vi "S2C_ExeScriptNextStep.vi"(8 "Error In":errorcluster, 11 "Q-Ref":refnum<queue>) -> (0 "Error Out":errorcluster)   [LabVIEW 2015]
doc: "Advances the executable script to the next step."
uses:
  Globals/S2C_Globals.vi
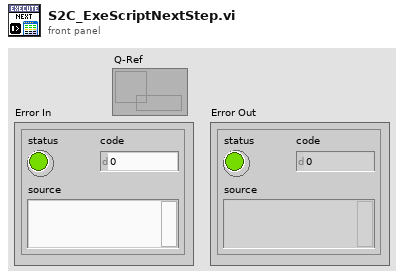
[diagram p1: front panel]
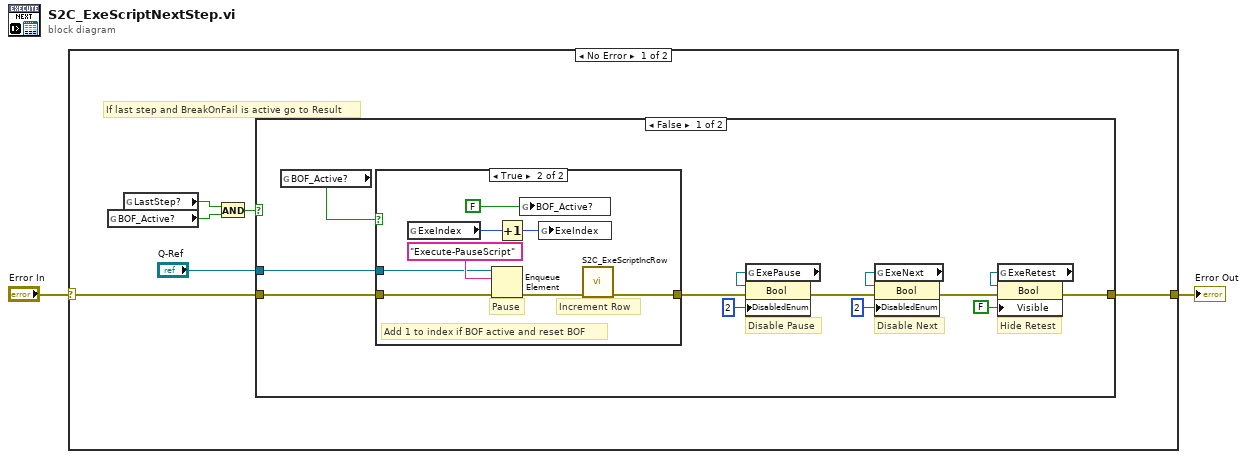
[diagram p0: block diagram]
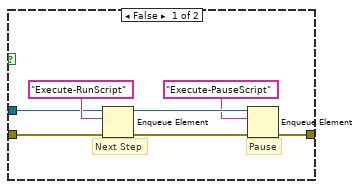
[diagram p2: hidden frame]
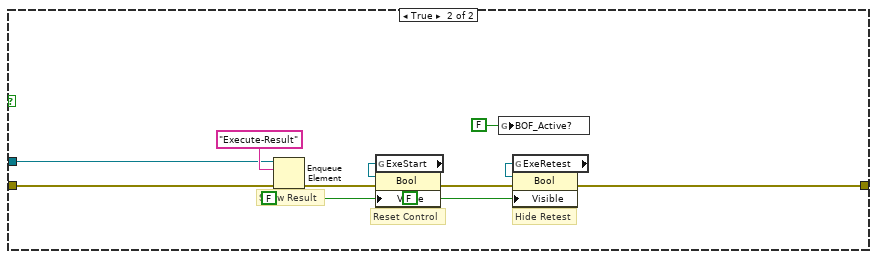
[diagram p3: hidden frame]
diagram:
  n1 = case shown="No Error" "Error In" {
    selector: "Error In" -> [w7 w48]
    tunnel: [w6 w48] -> w1
    frame No Error {
      # "If last step and BreakOnFail is active go to Result"
      n2 = global read "S2C_Globals.vi" "BOF_Active?"() -> (w4:bool)
      n3 = global read "S2C_Globals.vi" "LastStep?"() -> (w5:bool)
      n4 = And(x=w5, y=w4) -> (x .and. y?=w3:bool)
      n5 = case shown="False" w3 {
        tunnel: "Q-Ref" -> [w9 w42]
        tunnel: w7 -> [w10 w43]
        tunnel: [w11 w38] -> w6
        frame False {
          # "Hide Retest"
          # "Disable Pause"
          # "Disable Next"
          n6 = global read "S2C_Globals.vi" "BOF_Active?"() -> (w13:bool)
          n7 = case shown="True" w13 {
            tunnel: w10 -> [w24 w31]
            tunnel: [w23 w29] -> w12
            tunnel: w9 -> [w22 w33]
            frame False {
              # "Next Step"
              # "Pause"
              n8 = Enqueue Element(queue=w22, element="Execute-RunScript", error in (no error)=w24) -> (queue out=w27:refnum<queue>, error out=w26:errorcluster)  [unwired: 1 in, 1 out]
              n9 = Enqueue Element(queue=w27, element="Execute-PauseScript", error in (no error)=w26) -> (error out=w23:errorcluster)  [unwired: 1 in, 2 out]
            }
            frame True {
              # "Increment Row"
              # "Pause"
              # "Add 1 to index if BOF active and reset BOF"
              n10 = global read "S2C_Globals.vi" "ExeIndex"() -> (w35:i32)
              n11 = Enqueue Element(queue=w33, element="Execute-PauseScript", error in (no error)=w31) -> (error out=w30:errorcluster)  [unwired: 1 in, 2 out]
              n12 = Increment(x=w35) -> (x+1=w32:i32)
              n13 = global write "S2C_Globals.vi" "BOF_Active?"(FALSE ("BOF_Active?")) -> ()
              n14 = global write "S2C_Globals.vi" "ExeIndex"(w32) -> ()
              n15 = call "S2C_ExeScriptIncRow.vi"("Error In"=w30) -> ("Error Out"=w29:errorcluster)  [unwired: 10 in]
            }
          }
          n16 = global read "S2C_Globals.vi" "ExePause"() -> (w18:refnum<vi>)
          n17 = property on="Property Node" class="Bool"(reference=w18, error in=w12, "DisabledEnum"=u8 2) -> (error out=w17:errorcluster)  [unwired: 1 out]
          n18 = global read "S2C_Globals.vi" "ExeNext"() -> (w21:refnum<vi>)
          n19 = property on="Property Node" class="Bool"(reference=w21, error in=w17, "DisabledEnum"=u8 2) -> (error out=w15:errorcluster)  [unwired: 1 out]
          n20 = global read "S2C_Globals.vi" "ExeRetest"() -> (w16:refnum<vi>)
          n21 = property on="Property Node" class="Bool"(reference=w16, error in=w15, "Visible"=FALSE) -> (error out=w11:errorcluster)  [unwired: 1 out]
        }
        frame True {
          # "Hide Retest"
          # "Show Result"
          # "Reset Control"
          n22 = Enqueue Element(queue=w42, element="Execute-Result", error in (no error)=w43) -> (error out=w46:errorcluster)  [unwired: 1 in, 2 out]
          n23 = global read "S2C_Globals.vi" "ExeStart"() -> (w44:refnum<vi>)
          n24 = property class="Bool"(reference=w44, error in=w46, "Value"=FALSE) -> (error out=w39:errorcluster)  [unwired: 1 out]
          n25 = global write "S2C_Globals.vi" "BOF_Active?"(FALSE ("BOF_Active?")) -> ()
          n26 = global read "S2C_Globals.vi" "ExeRetest"() -> (w41:refnum<vi>)
          n27 = property on="Property Node" class="Bool"(reference=w41, error in=w39, "Visible"=FALSE) -> (error out=w38:errorcluster)  [unwired: 1 out]
        }
      }
    }
    frame Error {
    }
  }
  "Error Out" <- w1
